vi "Tusk.RegisterQueue.vi"(5 "Tusk in":refnum<class "Tusk.lvclass">, 7 "error in (no error)":errorcluster, 8 "Top Level?":bool, 11 "Name(Local)":string) -> (0 "error out":errorcluster, 3 "Tusk out":refnum<class "Tusk.lvclass">, 4 "Tusk out (copy)":refnum<class "Tusk.lvclass">, 6 "error out (copy)":errorcluster)   [LabVIEW 2018, in "Application.lvlib" / "Tusk.lvclass"]
uses:
  Tusk.lvclass
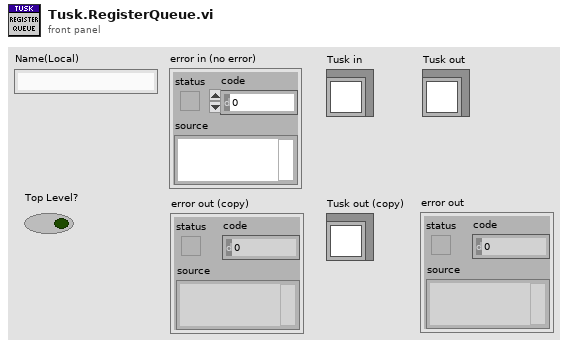
[diagram p1: front panel]
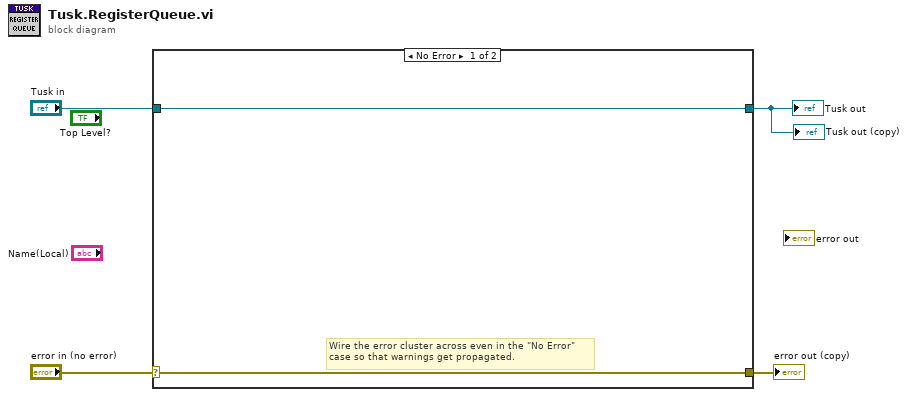
[diagram p0: block diagram]
diagram:
  n1 = case shown="No Error" "error in (no error)" {
    selector: "error in (no error)" -> [w6 w8]
    tunnel: [w6 w8] -> w3
    tunnel: [w5 w7] -> w1
    tunnel: "Tusk in" -> [w5 w7]
    frame No Error {
      # "Wire the error cluster across even in the \"No Error\"\ncase so that warnings get propagated."
    }
    frame Error {
    }
  }
  "error out (copy)" <- w3
  "Tusk out (copy)" <- w1
  "Tusk out" <- w1
